vi "Create Session Table.vi"(8 "error in (no error)":errorcluster, 11 "Test Results":T1 {"Analysis Results"."Linearity" format="%#4_2g"; "Analysis Results"."Repeatability" format="%#4_2g"; "Analysis Results"."Hysteresis" format="%#4_2g"; "Analysis Results"."Accuracy" format="%#4_2g"}) -> (0 "error out":errorcluster, 3 "Session Table":string[][](array[string]))   [LabVIEW 2026, in "Analysis.lvlib"]
uses:
  Analysis.lvlib
  Test Results.ctl
  Test Details.ctl
panel:
  # "Session Filters"
  # "%FS"
  # "%FS"
  # "%FS"
  # "%FS"
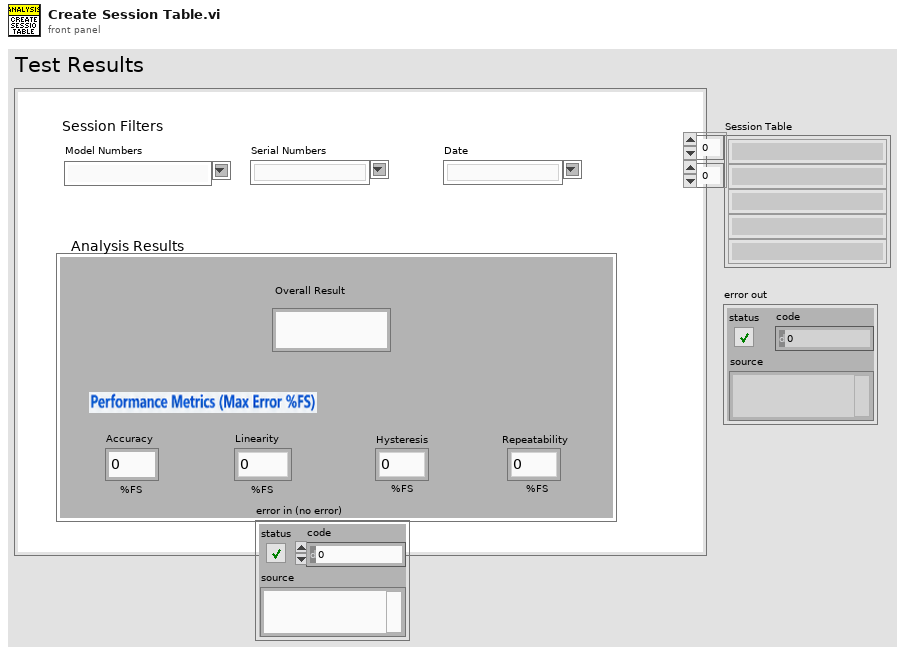
[diagram p1: front panel]
types:
  T1 = typedef "Analysis.lvlib/Test Results.ctl" = cluster{"Model Numbers":string, "Serial Numbers":string, "Date":string, "Analysis Results":T2}
  T2 = typedef "Analysis.lvlib/Test Details.ctl" = cluster{"Accuracy":dbl, "Hysteresis":dbl, "Repeatability":dbl, "Linearity":dbl, "Overall Result":string}
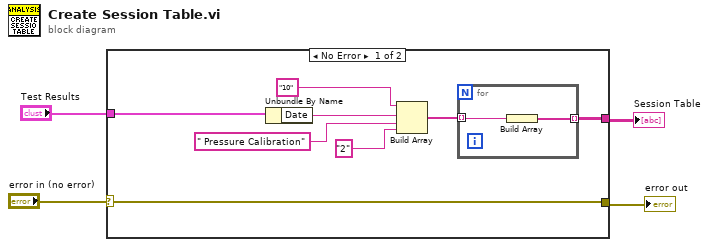
[diagram p0: block diagram]
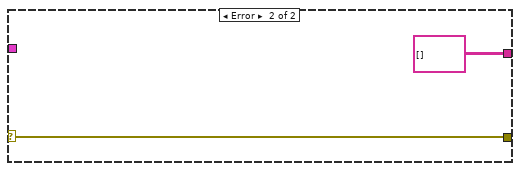
[diagram p2: hidden frame]
diagram:
  n1 = case shown="No Error" "error in (no error)" {
    selector: "error in (no error)" -> [w12 w16]
    tunnel: [w12 w16] -> w3
    tunnel: [w6 string[][] []] -> w2
    tunnel: "Test Results" -> [w5 _]
    frame No Error {
      n2 = Unbundle By Name(w5) -> ("Date"=w11:string)
      n3 = Build Array("10" ("element"), w11, " Pressure Calibration" ("element"), "2" ("element")) -> (w7:string[])
      n4 = for {
        tunnel: w7 -> [w14] mode=indexing
        tunnel: [w13] -> w6 mode=indexing
        n5 = Build Array(w14) -> (w13:string[])
      }
    }
    frame Error {
    }
  }
  "Session Table" <- w2
  "error out" <- w3
